vi "getAdditionalDataFromXMLNative.vi"(8 "error in (no error)":errorcluster, 10 "eventXML":refnum<k20>, 11 "rf in":refnum<class "rf.lvclass">) -> (0 "error out":errorcluster, 2 "eventXML out":refnum<k20>, 3 "rf out":refnum<class "rf.lvclass">)   [LabVIEW 2009, in "Tools.lvlib" / "Scripting.lvlib" / "rf.lvclass"]
uses:
  rf.lvclass
  RfArray/rfArray.lvclass
  <vilib>/xml/Close Reference(Node).vi
  rf.lvclass/rf.ctl
  <vilib>/xml/NI_XML.lvlib
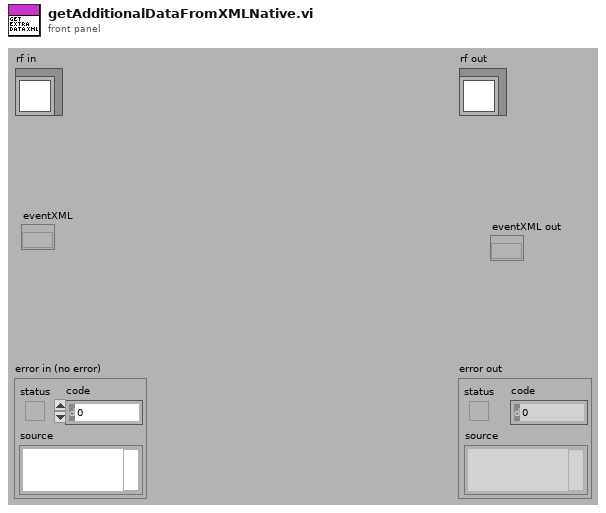
[diagram p1: front panel]
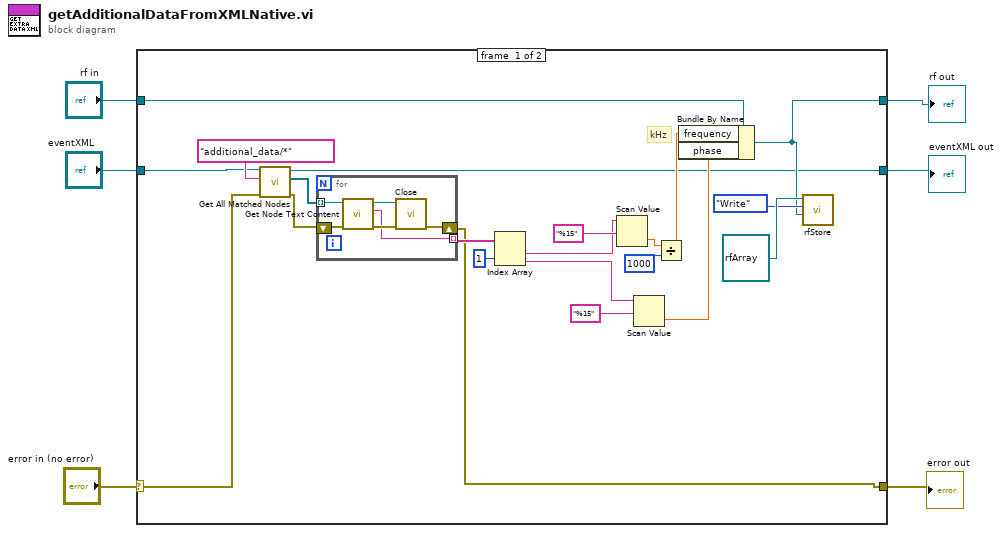
[diagram p0: block diagram]
diagram:
  n1 = case shown="No Error" "error in (no error)" {
    selector: "error in (no error)" -> [w11 w34]
    tunnel: [w9 w34] -> w5
    tunnel: [w18 w35] -> w4
    tunnel: "rf in" -> [w19 w35]
    tunnel: "eventXML" -> [w12 _]
    tunnel: [w10 _] -> w1
    frame #0 {
      # "kHz"
      n2 = call <vilib>:"Get All Matched Nodes.vi"("error in (no error)"=w11, "XPath expression"="additional_data/*", "node in"=w12) -> ("error out"=w17:errorcluster, "node result array"=w15:refnum<k20>[], "node out"=w10:refnum<k20>)  [unwired: 6 in]
      n3 = for {
        tunnel: w15 -> [w30] mode=indexing
        tunnel: [w29] -> w14 mode=indexing
        shift-right: [w28] -> w9
        shift-left: w17 -> [w31]
        n4 = call <vilib>:"Get Node Text Content.vi"("error in (no error)"=w31, "node in"=w30) -> ("error out"=w32:errorcluster, "node text"=w29:string, "node out"=w33:refnum<k20>)  [unwired: 7 in]
        n5 = call-poly <vilib>:"Close.vi"("error in (no error)"=w32, "node"=w33) -> ("error out"=w28:errorcluster)  [unwired: 7 in]
      }
      n6 = Index Array(array=w14, index #2=1 ("index")) -> (element #1=w8:string, element #2=w7:string)  [unwired: 1 in]
      n7 = Scan Value(string=w8, format string="%15") -> (value=w26:dbl)  [unwired: 1 in, 1 out]
      n8 = Scan Value(string=w7, format string="%15") -> (value=w22:dbl)  [unwired: 1 in, 1 out]
      n9 = Divide(x=w26, y=1000) -> (x/y=w24:dbl)
      n10 = Bundle By Name(cluster=w19, "frequency"=w24, "phase"=w22) -> (w18:refnum<class "rf.lvclass">)
      n11 = call "rfStore.vi"("rf.lvclass"=w18, "action"=enum16{"Write", "Read"}."Write", "rfArray in"=refnum<class "rfArray.lvclass"> refnum ("Tools.lvlib:Scripting.lvlib:rfArray.lvclass")) -> ()  [unwired: 5 in, 4 out]
    }
    frame #1 {
    }
  }
  "error out" <- w5
  "rf out" <- w4
  "eventXML out" <- w1
